vi "LoadSegmentOptions.vi"(7 "Item Ref in":T1 format="%.0x", 8 "error in (no error)":errorcluster, 9 "Segment by":refnum<vi>, 10 "Segment every":refnum<vi>, 11 "Boolean in":refnum<vi>) -> (0 "error out":errorcluster, 3 "Item Ref out":T1 format="%.0x")   [LabVIEW 2024, in "Embedded TDMS Logger System Explorer.lvlib"]
doc: "Load the segmentation options defined in the System Definition file for population into the Main Page VI."
uses:
  Embedded TDMS Logger System Explorer.lvlib
  <vilib>/NI VeriStand/Custom Device API/Custom Device Item Ref.ctl
  <vilib>/NI VeriStand/Custom Device API/Get Item Property (Double).vi
  <vilib>/NI VeriStand/Custom Device API/Set Item Property (Double).vi
  <vilib>/NI VeriStand/Custom Device API/Get Item Property (Boolean).vi
  <vilib>/NI VeriStand/Custom Device API/Set Item Property (Boolean).vi
  <vilib>/NI VeriStand/Custom Device API/Get Item Property (U16).vi
  <vilib>/NI VeriStand/Custom Device API/Set Item Property (U16).vi
  <vilib>/NI VeriStand/Custom Device API/Custom Device API.lvlib
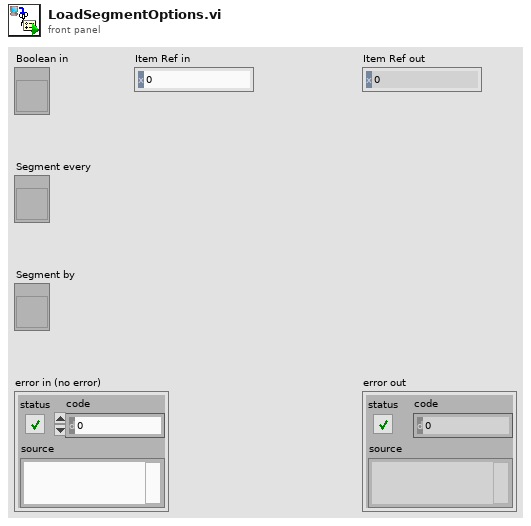
[diagram p1: front panel]
types:
  T1 = typedef "Custom Device API.lvlib/Custom Device Item Ref.ctl" = u64
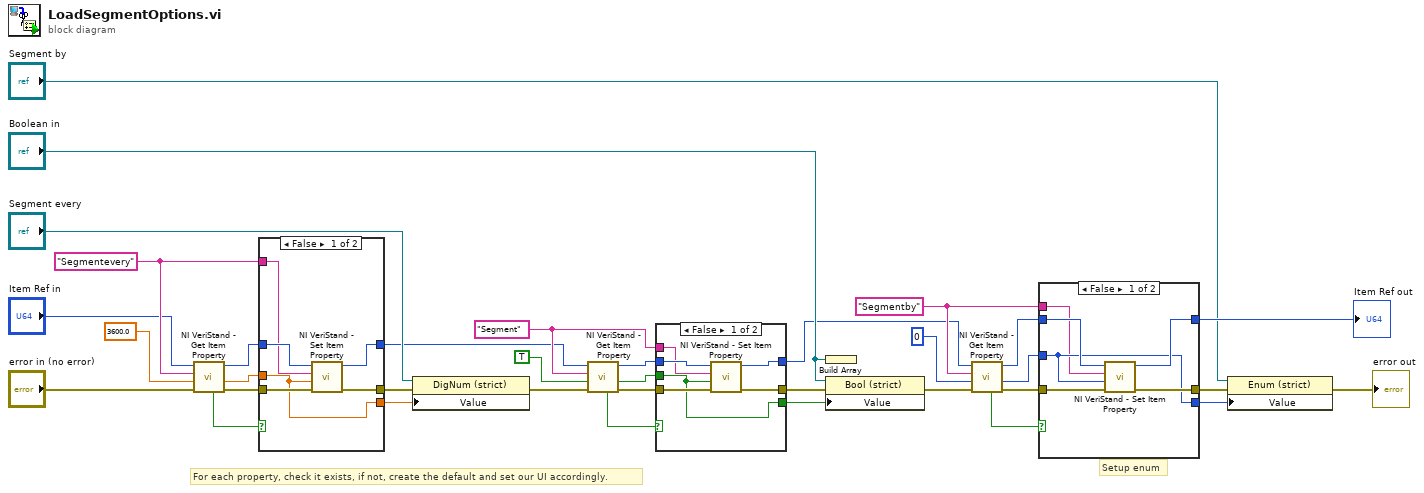
[diagram p0: block diagram]
diagram:
  w7 = "Segmentevery"
  w14 = "Segment"
  w33 = "Segmentby"
  # "For each property, check it exists, if not, create the default and set our UI accordingly."
  # "Setup enum"
  n1 = call-poly <vilib>:"NI VeriStand - Get Item Property.vi"("error in (no error)"="error in (no error)", "Default Value"=3600.0 ("Numeric"), "Property Name"=w7, "Item Ref in"="Item Ref in") -> ("error out"=w11:errorcluster, "Value"=w12:dbl, "Item Ref out"=w10:T1, "Found?"=w13:bool)  [unwired: 4 in]
  n2 = case shown="False" w13 {
    tunnel: w10 -> [w41 w44]
    tunnel: w11 -> [w40 w43]
    tunnel: [w39 w43] -> w9
    tunnel: [w38 w44] -> w2
    tunnel: w12 -> [w37 w42]
    tunnel: [w37 w42] -> w5
    tunnel: w7 -> [w36 _]
    frame False {
      n3 = call-poly <vilib>:"NI VeriStand - Set Item Property.vi"("error in (no error)"=w40, "Value"=w37, "Property Name"=w36, "Item Ref in"=w41) -> ("error out"=w39:errorcluster, "Item Ref out"=w38:T1)  [unwired: 5 in, 1 out]
    }
    frame True {
    }
  }
  n4 = property class="DigNum (strict)"(reference="Segment every", error in=w9, "Value"=w5) -> (error out=w1:errorcluster)  [unwired: 1 out]
  n5 = call-poly <vilib>:"NI VeriStand - Get Item Property.vi"("error in (no error)"=w1, "Default Value"=TRUE, "Property Name"=w14, "Item Ref in"=w2) -> ("error out"=w21:errorcluster, "Value"=w18:bool, "Item Ref out"=w22:T1, "Found?"=w16:bool)  [unwired: 4 in]
  n6 = case shown="False" w16 {
    tunnel: w22 -> [w50 w53]
    tunnel: w21 -> [w49 w52]
    tunnel: [w48 w52] -> w20
    tunnel: [w47 w53] -> w19
    tunnel: w18 -> [w46 w51]
    tunnel: [w46 w51] -> w17
    tunnel: w14 -> [w45 _]
    frame False {
      n7 = call-poly <vilib>:"NI VeriStand - Set Item Property.vi"("error in (no error)"=w49, "Value"=w46, "Property Name"=w45, "Item Ref in"=w50) -> ("error out"=w48:errorcluster, "Item Ref out"=w47:T1)  [unwired: 5 in, 1 out]
    }
    frame True {
    }
  }
  n8 = Build Array("Boolean in") -> ()  [unwired: 1 out]
  n9 = property class="Bool (strict)"(reference="Boolean in", error in=w20, "Value"=w17) -> (error out=w24:errorcluster)  [unwired: 1 out]
  n10 = call-poly <vilib>:"NI VeriStand - Get Item Property.vi"("error in (no error)"=w24, "Default Value"=u16 0, "Property Name"=w33, "Item Ref in"=w19) -> ("error out"=w27:errorcluster, "Value"=w25:u16, "Item Ref out"=w26:T1, "Found?"=w28:bool)  [unwired: 4 in]
  n11 = case shown="False" w28 {
    tunnel: [w59 w62] -> w34
    tunnel: w26 -> [w58 w62]
    tunnel: [w57 w61] -> w29
    tunnel: w27 -> [w56 w61]
    tunnel: w25 -> [w55 w60]
    tunnel: [w55 w60] -> w32
    tunnel: w33 -> [w54 _]
    frame False {
      n12 = call-poly <vilib>:"NI VeriStand - Set Item Property.vi"("error in (no error)"=w56, "Value"=w55, "Property Name"=w54, "Item Ref in"=w58) -> ("error out"=w57:errorcluster, "Item Ref out"=w59:T1)  [unwired: 5 in, 1 out]
    }
    frame True {
    }
  }
  "Item Ref out" <- w34
  n13 = property class="Enum (strict)"(reference="Segment by", error in=w29, "Value"=w32) -> (error out=→"error out":errorcluster)  [unwired: 1 out]
